vi "PH_HamamatsuCamera.configure Parameter.vi"(0 "i ref in":refnum<vi>, 1 "Cam Handle in":i32, 4 "Cam Error in":errorcluster, 5 "error in (no error)":errorcluster) -> (14 "VI out":refnum<vi>, 15 "Cam Handle out":i32, 18 "Cam Error out":errorcluster, 19 "error out":errorcluster)   [LabVIEW 2014, in "PH_HamamatsuCamera.lvlib"]
uses:
  PH_HamamatsuCamera.lvlib
  PH_Cam_BaseClass/PH_Cam_BaseClass.lvlib
panel:
  in  "Parameter Dummy":u32(ring)=4215968 items=["SENSOR MODE"=4212128, "CCD MODE"=4212384, "READOUT MODE"=4211872, "ACTIVE VIEW INDEX"=4343136, "BITS PER CHANNEL"=4342976, "IMAGE PIXEL TYPE"=4343296, "BINNING"=4215968, "EXPOSURE TIME"=2049184, "CONTRAST GAIN"=3163312, "CONTRAST OFFSET"=3163328, "LIGHT MODE"=2114720, "SENSITIVITY"=2114992, "PHOTON IMAGING MODE"=2115200, "HIGH DYNAMIC RANGE MODE"=3163360, "WHITE BALANCE"=3163568, "TEMPERATURE"=2115232, "TEMPERATURE TARGET"=2115264, "SENSOR COOLER FAN"=2115296, "LINEBUNDLE HEIGHT"=4212192, "MECHANICAL SHUTTER"=2115488, "BACK FOCUS POSITION"=8422304, "TRIGGER CONNECTOR"=1066432, "TRIGGER SOURCE"=1066144, "OUTPUT TRIGGER SOURCE"=1852576, "TRIGGER GLOBAL EXPOSURE"=2049680, "FIRST TRIGGER BEHAVIOR"=2049696, "CHANNEL SYNC"=1852352, "READOUT DIRECTION"=4211904, "PRE HSYNC COUNT"=1852704, "INTERNAL LINE SPEED"=4191408, "INTERNAL LINE INTERVAL"=4191424]
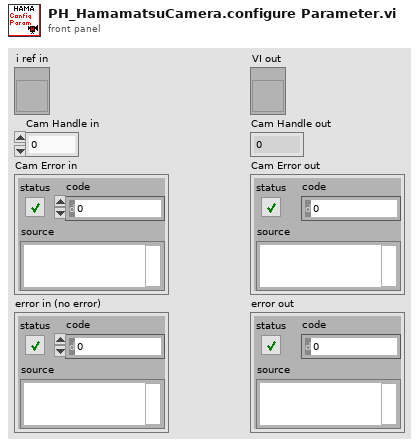
[diagram p1: front panel]
types:
  T1 = typedef "PH_HamamatsuCamera.lvlib/PH_HamamatsuCamera.i attribute.ctl" = cluster{"Gui Refs":cluster{"Camera Details":refnum<vi>, "ROI":refnum<vi>, "Set ROI to Maximum":refnum<vi>, "Trigger Parameters":refnum<vi>, "Brightness":refnum<vi>, "Shutter":refnum<vi>, "Gain":refnum<vi>, "Trigger Timeout":refnum<vi>, "Trigger Polarity":refnum<vi>, "Trigger Mode":refnum<vi>, "Parameters":refnum<vi>, "Set Cam Parameter":refnum<vi>, "Parameter to set":refnum<vi>, "Value to set":refnum<vi>}, "Cam":cluster{"Handle":i32, "Details":cluster{"Model":string, "Camera ID":string, "Firmware":string}, "Buffer Info":cluster{"height":u32, "width":u32, "datatype":u32}}, "H Offset":cluster{"Value":i32, "Minimum":i32, "Maximum":i32, "Increment":i32}, "V Offset":cluster{"Value":i32, "Minimum":i32, "Maximum":i32, "Increment":i32}, "H Width":cluster{"Value":i32, "Minimum":i32, "Maximum":i32, "Increment":i32}, "V Width":cluster{"Value":i32, "Minimum":i32, "Maximum":i32, "Increment":i32}, "Trigger Parameters":T2, "Trigger Timeout":u32, "Parameters":T3[], "Indicees Cam Parameters":cluster{"Brightness":i32, "Shutter":i32, "Gain":i32}, "Wanted Values":cluster{"Trigger Settings":T2[], "ROI":T4[], "Parameter":cluster{"Name":string, "Value":dbl}[]}}
  T2 = typedef "PH_HamamatsuCamera.lvlib/PH_HamamatsuCamera.Trigger Parameter.ctl" = cluster{"Mode":u32, "Polarity":u32, "Times":u32, "Delay":dbl}
  T3 = typedef "PH_HamamatsuCamera.lvlib/PH_HamamatsuCamera.Parameter Set.ctl" = cluster{"Parameter":string, "Value":dbl, "Writable":bool, "Range":cluster{"min":dbl, "max":dbl, "step":dbl}, "Default":dbl, "Value Names":cluster{"Name":string, "Value":dbl}[], "Text Values":bool}
  T4 = typedef "PH_HamamatsuCamera.lvlib/PH_HamamatsuCamera.ROI.ctl" = cluster{"Horizontal Offset":i32, "Vertical Offset":i32, "Horizontal Width":i32, "Vertical Width":i32}
  T5 = typedef "PH_Cam_BaseClass.lvlib/PH_Cam_BaseClass.Settings.ctl" = cluster{"Cam ID":string, "Gain":dbl, "Brightness":dbl, "Shutter":dbl, "Mode":i32}
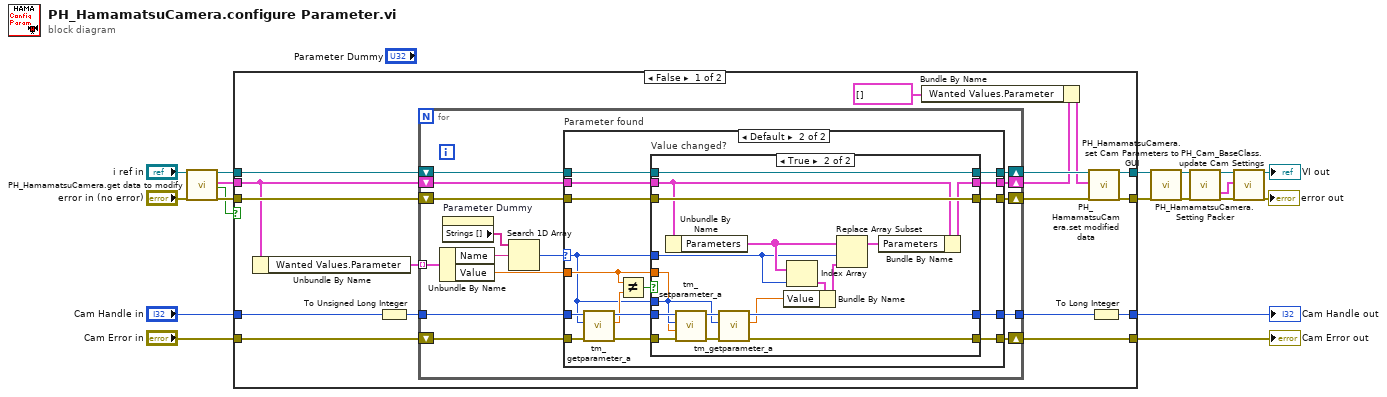
[diagram p0: block diagram]
diagram:
  n1 = call "PH_HamamatsuCamera.get data to modify.vi"("i ref in"="i ref in", "error in (no error)"="error in (no error)") -> ("i ref out"=w13:refnum<vi>, "i attribute"=w12:T1, "timed out"=w9:bool, "error out"=w15:errorcluster)  [unwired: 14 in]
  n2 = case shown="False" w9 {
    tunnel: [w35 w96] -> w19
    tunnel: "Cam Handle in" -> [w34 w97]
    tunnel: "Cam Error in" -> [w31 w96]
    tunnel: w15 -> [w30 w98]
    tunnel: w13 -> [w29 w99]
    tunnel: w12 -> [w24 _]
    tunnel: [w28 w97] -> w11
    tunnel: [w20 w98] -> w10
    tunnel: [w25 w99] -> w3
    frame False {
      n3 = Unbundle By Name(w24) -> ("Wanted Values.Parameter"=w27:cluster{"Name":string, "Value":dbl}[])
      n4 = To Unsigned Long Integer(number=w34) -> (unsigned 32bit integer=w32:u32)
      n5 = for {
        tunnel: w32 -> [w44]
        shift-right: [w51] -> w35
        shift-left: w31 -> [w45]
        tunnel: [w50] -> w33
        shift-right: [w48] -> w26
        shift-left: w29 -> [w49]
        shift-right: [w46] -> w36
        shift-left: w30 -> [w47]
        tunnel: w27 -> [w42] mode=indexing
        shift-right: [w39] -> w23
        shift-left: w24 -> [w40]
        n6 = Unbundle By Name(w42) -> ("Name"=w41:string, "Value"=w38:dbl)
        n7 = property on="Parameter Dummy" class="Ring (strict)"() -> ("Strings []"=w43:string[])  [unwired: 2 in, 2 out]
        n8 = Search 1D Array(1D array=w43, element=w41) -> (index of element=w37:i32)  [unwired: 1 in]
        n9 = case "Parameter found" shown="Default" w37 {
          selector: w37 -> [_ w57]
          tunnel: [w52 w72] -> w51
          tunnel: [w53 w70] -> w50
          tunnel: w49 -> [w56 w69]
          tunnel: [w56 w68] -> w48
          tunnel: w47 -> [w54 w67]
          tunnel: [w54 w66] -> w46
          tunnel: w45 -> [w52 w65]
          tunnel: w44 -> [w53 w63]
          tunnel: w40 -> [w55 w61]
          tunnel: [w55 w60] -> w39
          tunnel: w38 -> [_ w59]
          frame -1 {
          }
          frame Default {
            n10 = call <userlib>:"tm_getparameter_a.vi"("error in (no error)"=w65, "Parameter"=w57, "Handle in"=w63) -> ("error out"=w64:errorcluster, "Value out"=w58:dbl, "Handle out"=w62:u32)  [unwired: 6 in]
            n11 = Not Equal?(x=w59, y=w58) -> (x != y?=w71:bool)
            n12 = case "Value changed?" shown="True" w71 {
              tunnel: w64 -> [w77 w95]
              tunnel: w62 -> [w76 w94]
              tunnel: w57 -> [_ w89]
              tunnel: [w77 w90] -> w72
              tunnel: [w76 w93] -> w70
              tunnel: w69 -> [w75 w88]
              tunnel: [w75 w88] -> w68
              tunnel: w67 -> [w74 w87]
              tunnel: [w74 w87] -> w66
              tunnel: w59 -> [_ w79]
              tunnel: w57 -> [_ w82]
              tunnel: w61 -> [w73 w85]
              tunnel: [w73 w86] -> w60
              frame False {
              }
              frame True {
                n13 = Unbundle By Name(w85) -> ("Parameters"=w83:T3[])
                n14 = call <userlib>:"tm_setparameter_a.vi"("error in (no error)"=w95, "Value in"=w79, "Parameter"=w89, "Handle in"=w94) -> ("error out"=w91:errorcluster, "Handle out"=w92:u32)  [unwired: 6 in]
                n15 = call <userlib>:"tm_getparameter_a.vi"("error in (no error)"=w91, "Parameter"=w89, "Handle in"=w92) -> ("error out"=w90:errorcluster, "Value out"=w78:dbl, "Handle out"=w93:u32)  [unwired: 6 in]
                n16 = Index Array(array=w83, index=w82) -> (element=w81:T3)
                n17 = Bundle By Name(cluster=w81, "Value"=w78) -> (w80:T3)
                n18 = Replace Array Subset(array=w83, new element=w80, index=w82) -> (w84:T3[])
                n19 = Bundle By Name(cluster=w85, "Parameters"=w84) -> (w86:T1)
              }
            }
          }
        }
      }
      n20 = Bundle By Name(cluster=w23, "Wanted Values.Parameter"=cluster{"Name":string, "Value":dbl}[] []) -> (w21:T1)
      n21 = call "PH_HamamatsuCamera.set modified data.vi"("i ref in"=w26, "i attribute"=w21, "error in (no error)"=w36) -> ("i ref out"=w25:refnum<vi>, "error out"=w20:errorcluster)  [unwired: 15 in]
      n22 = To Long Integer(number=w33) -> (32bit integer=w28:i32)
    }
    frame True {
    }
  }
  "Cam Error out" <- w19
  "Cam Handle out" <- w11
  n23 = call "PH_HamamatsuCamera.set Cam Parameters to GUI.vi"("i ref in"=w3, "error in (no error)"=w10) -> ("VI out"=w2:refnum<vi>, "error out"=w5:errorcluster)  [unwired: 16 in]
  n24 = call "PH_HamamatsuCamera.Setting Packer.vi"("i ref in"=w2, "error in (no error)"=w5) -> ("i ref out"=w7:refnum<vi>, "Cam Settings"=w6:T5, "error out"=w8:errorcluster)  [unwired: 15 in]
  n25 = call "PH_Cam_BaseClass.update Cam Settings.vi"("VI in"=w7, "Cam Settings In"=w6, "error in (no error)"=w8) -> ("VI out"=→"VI out":refnum<vi>, "error out"=→"error out":errorcluster)  [unwired: 15 in]
